vi "Close.vi"(8 "error in (no error)":errorcluster, 11 "Monkey in":refnum<class "Monkey.lvclass">) -> (0 "error out":errorcluster, 3 "Monkey out":refnum<class "Monkey.lvclass">)   [LabVIEW 2020, in "Monkey.lvlib" / "Monkey.lvclass"]
uses:
  Monkey.lvclass
  C:/Users/aegis/Documents/CIRCUS/TALOS/TALOS_PPL.lvlibp/Ancestor/Ancestor/Ancestor.lvclass
  TALOS/TALOS_PPL.lvlibp/Ancestor/Ancestor/Read ID.vi
  TALOS/TALOS_PPL.lvlibp/Support VIs/Global Constants.vi
  TALOS/TALOS_PPL.lvlibp/Father of all uServices/Father of all uServices/Father of all uServices.lvclass
  TALOS/TALOS_PPL.lvlibp
  C:/Users/aegis/Documents/CIRCUS/TALOS/TALOS_PPL.lvlibp/Father of all uServices/Father of all uServices/Father of all uServices.lvclass
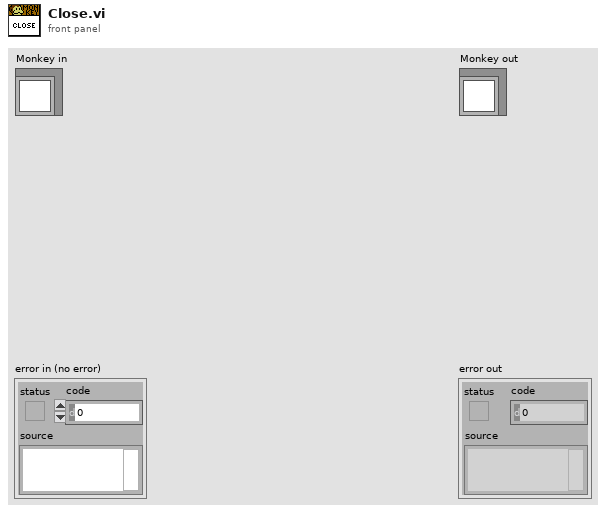
[diagram p1: front panel]
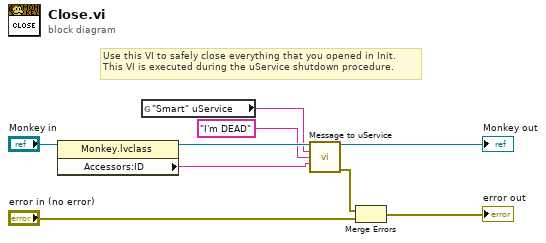
[diagram p0: block diagram]
diagram:
  # "Use this VI to safely close everything that you opened in Init.\nThis VI is executed during the uService shutdown procedure."
  n1 = property class="Monkey.lvclass"(reference="Monkey in") -> (reference out=w8:refnum<class "Monkey.lvclass">, "Accessors:ID"=w6:string)  [unwired: 1 in, 1 out]
  n2 = global read "Global Constants.vi" "\"Smart\" uService"() -> (w1:string)
  n3 = call "Message to uService.vi"("Father of all uServices in"=w8, "uService ID"=w1, "Message"="I'm DEAD", "Data"=w6) -> ("Father of all uServices out"=→"Monkey out":refnum<class "Monkey.lvclass">, "error out"=w3:errorcluster)  [unwired: 10 in]
  n4 = Merge Errors(w3, "error in (no error)") -> (→"error out":errorcluster)
